vi "Get all Object Item Offsets.vi"(8 "error in (no error)":errorcluster, 10 "Offset":i32, 11 "JSON":string) -> (0 "error out":errorcluster, 1 "Items":T1[](array[typedef]), 2 "Offset past Object":i32)   [LabVIEW 2017, in "JSONtext.lvlib"]
uses:
  JSONtext.lvlib
  Parsing/Found Items.ctl
  Parsing/Parsing State.ctl
  Parsing/Advance past Number.vi
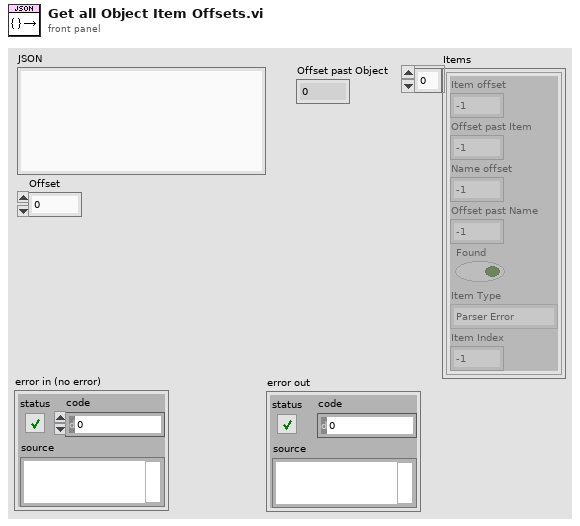
[diagram p1: front panel]
types:
  T1 = typedef "JSONtext.lvlib/Found Items.ctl" = cluster{"Item offset":i32, "Offset past Item":i32, "Name offset":i32, "Offset past Name":i32, "Found":bool, "Item Type":T2, "Item Index":i32}
  T2 = typedef "JSONtext.lvlib/Parsing State.ctl" = enum16{"Parser Error", "Object", "Array", "String", "Number/Other", "Leading Whitespace", "Object end", "Array end", "Value end"}
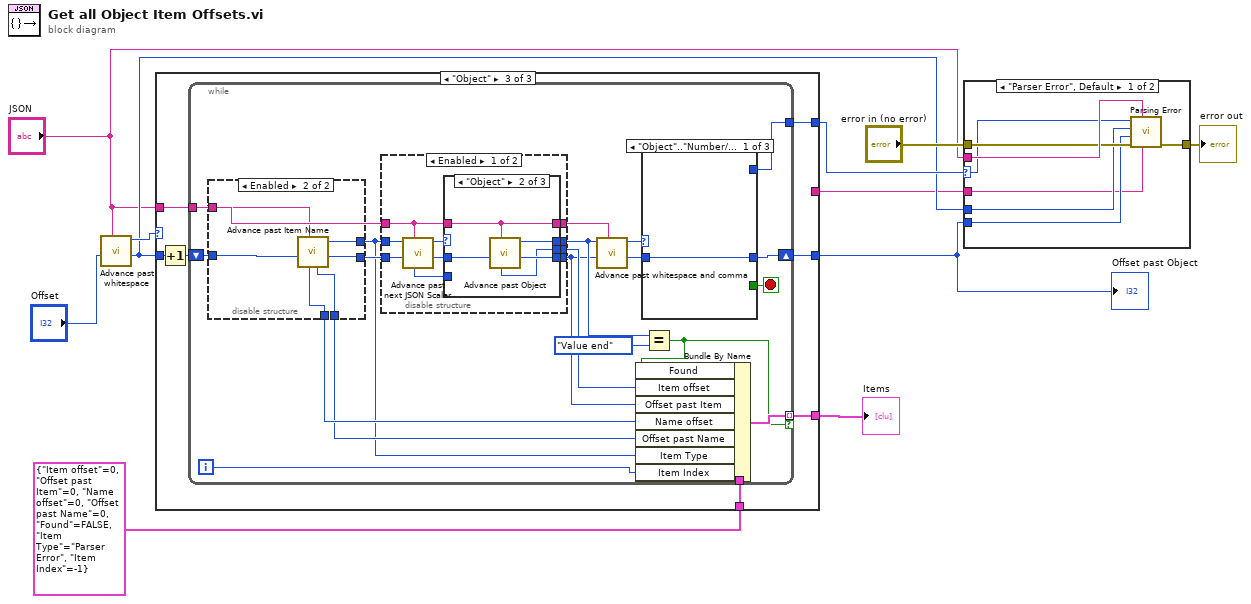
[diagram p0: block diagram]
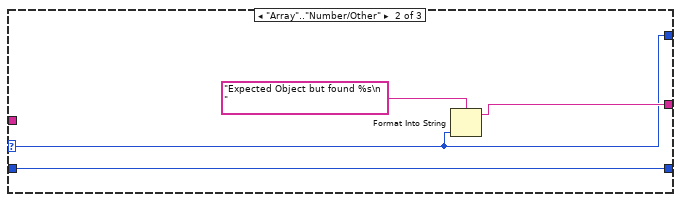
[diagram p3: hidden frame]
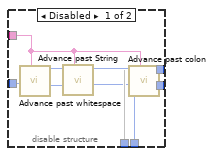
[diagram p4: hidden frame]
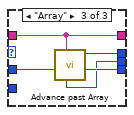
[diagram p6: hidden frame]
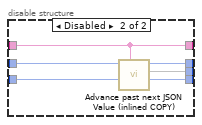
[diagram p7: hidden frame]
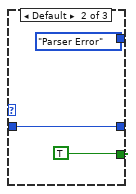
[diagram p8: hidden frame]
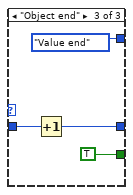
[diagram p9: hidden frame]
diagram:
  n1 = call "Advance past whitespace.vi"("JSON"="JSON", "Offset"="Offset") -> ("Offset of first non-whitespace"=w5:i32, "Parser State"=w10:T2)  [unwired: 8 in]
  n2 = case shown="\"Object\"" w10 {
    selector: w10 -> [w13 w14 _]
    tunnel: [w13 w14 w24] -> w6
    tunnel: w5 -> [w12 w17 w22]
    tunnel: "JSON" -> [_ _ w21]
    tunnel: [w12 w17 w20] -> w7
    tunnel: [_ _ w19] -> w3
    tunnel: T1 {"Item offset"=0, "Offset past Item"=0, "Name offset"=0, "Offset past Name"=0, "Found"=FALSE, "Item Type"=enum."Parser Error", "Item Index"=-1} -> [_ _ w18]
    tunnel: [_ w15 _] -> w1
    frame "Parser Error", Default {
    }
    frame "Array".."Number/Other" {
      n3 = Format Into String(format string="Expected Object but found %s\n " ("initial string"), w14) -> (resulting string=w15:string)  [unwired: 2 in, 1 out]
    }
    frame "Object" {
      n4 = Increment(x=w22) -> (x+1=w23:i32)
      n5 = while {
        shift-right: [w42] -> w20
        shift-left: w23 -> [w39]
        tunnel: w21 -> [w36]
        tunnel: [w40] -> w24
        tunnel: [w31] -> w19 mode=indexing if=w30
        tunnel: w18 -> [w27]
        i -> [w25]
        stop <- w41 stop-if-true
        n6 = disable-structure shown="Enabled" {
          disable-tunnel: w39 -> [w52 w57]
          disable-tunnel: [w49 w59] -> w26
          disable-tunnel: [w48 w58] -> w37
          disable-tunnel: w36 -> [w47 w56]
          disable-tunnel: [w46 w55] -> w29
          disable-tunnel: [w45 w54] -> w28
          frame Disabled {
            n7 = call "Advance past whitespace.vi"("JSON"=w47, "Offset"=w52) -> ("Offset of first non-whitespace"=w51:i32, "Parser State"=w50:T2)  [unwired: 8 in]
            n8 = call "Advance past String.vi"("JSON"=w47, "Offset"=w51, "State in"=w50) -> ("Offset past match"=w45:i32, 2:w46, "State"=w53:T2)  [unwired: 5 in, 1 out]
            n9 = call "Advance past colon.vi"("JSON"=w47, "Offset"=w45, "State"=w53) -> ("index"=w48:i32, "State"=w49:T2)  [unwired: 7 in]
          }
          frame Enabled {
            n10 = call "Advance past Item Name.vi"("JSON"=w56, "Offset"=w57) -> ("Offset past colon"=w58:i32, "State"=w59:T2, "Offset past Name"=w54:i32, "Name start out"=w55:i32)  [unwired: 6 in]
          }
        }
        n11 = disable-structure shown="Enabled" {
          disable-tunnel: [w69 w84] -> w38
          disable-tunnel: w26 -> [w67 w86]
          disable-tunnel: w37 -> [w66 w85]
          disable-tunnel: w36 -> [w64 w84]
          disable-tunnel: [w63 w87] -> w35
          disable-tunnel: [w62 w88] -> w33
          disable-tunnel: [w61 w89] -> w32
          frame Enabled {
            n12 = call "Advance past next JSON Scaler.vi"("JSON"=w64, "Offset"=w66, "Parser State in"=w67) -> ("Offset Past"=w65:i32, "Parser State"=w68:T2, "Value start"=w60:i32)  [unwired: 6 in]
            n13 = case shown="\"Object\"" w68 {
              selector: w68 -> [w72 _ _]
              tunnel: w65 -> [w71 w78 w83]
              tunnel: [w72 w77 w82] -> w63
              tunnel: [w71 w76 w81] -> w61
              tunnel: w64 -> [w73 w75 w80]
              tunnel: [w73 w75 w80] -> w69
              tunnel: [w70 w74 w79] -> w62
              tunnel: w60 -> [w70 _ _]
              frame Default {
              }
              frame "Object" {
                n14 = call "Advance past Object.vi"("JSON"=w75, "Offset"=w78) -> ("Offset past Object"=w76:i32, "State"=w77:T2, "Object Start"=w74:i32)  [unwired: 7 in]
              }
              frame "Array" {
                n15 = call "Advance past Array.vi"("JSON"=w80, "Offset"=w83) -> ("Offset past Array"=w81:i32, "State"=w82:T2, "Array Start"=w79:i32)  [unwired: 6 in, 1 out]
              }
            }
          }
          frame Disabled {
            n16 = call "Advance past next JSON Value (inlined COPY).vi"("JSON"=w84, "Offset"=w85, "State"=w86) -> ("Offset"=w89:i32, 2:w88, "State"=w87:T2)  [unwired: 3 in, 3 out]
          }
        }
        n17 = call "Advance past whitespace and comma.vi"("JSON"=w38, "Offset"=w32, "State in"=w35) -> ("Offset past match"=w44:i32, "State"=w43:T2)  [unwired: 7 in]
        n18 = case shown="\"Object\"..\"Number/Other\"" w43 {
          tunnel: [_ TRUE TRUE] -> w41
          tunnel: [_ Parsing_State."Parser Error" Parsing_State."Value end"] -> w40
          tunnel: w44 -> [w90 w91 w95]
          tunnel: [w90 w91 w94] -> w42
          frame "Object".."Number/Other" {
          }
          frame Default {
          }
          frame "Object end" {
            n19 = Increment(x=w95) -> (x+1=w94:i32)
          }
        }
        n20 = Equal?(x=w35, y=Parsing_State."Value end") -> (x = y?=w30:bool)
        n21 = Bundle By Name(cluster=w27, "Found"=w30, "Item offset"=w33, "Offset past Item"=w32, "Name offset"=w29, "Offset past Name"=w28, "Item Type"=w26, "Item Index"=w25) -> (w31:T1)
      }
    }
  }
  "Offset past Object" <- w7
  "Items" <- w3
  n22 = case shown="\"Parser Error\", Default" w6 {
    selector: w6 -> [w99 _]
    tunnel: "JSON" -> [w104 _]
    tunnel: "error in (no error)" -> [w103 w105]
    tunnel: [w102 w105] -> w9
    tunnel: w5 -> [w101 _]
    tunnel: w7 -> [w100 _]
    tunnel: w1 -> [w98 _]
    frame "Parser Error", Default {
      n23 = call "Parsing Error.vi"("initial string"=w98, "JSON"=w104, "error in (no error)"=w103, "Offset past match"=w100, "Value start"=w101, "State"=w99) -> ("error out"=w102:errorcluster)  [unwired: 5 in]
    }
    frame "Value end" {
    }
  }
  "error out" <- w9
